vi "Global_Drive_Turn_sens.vi"() -> ()   [LabVIEW 2017]
panel:
  in  "Height Gear Max Turn Sens":dbl
  in  "Low Gear Max Turn Sens":dbl
  in  "Height Gear Min Turn Sens":dbl
  in  "Low Gear Min Turn Sens":dbl
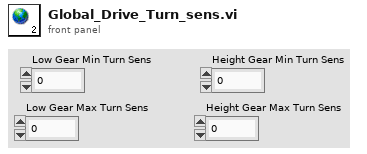
[diagram p1: front panel]
diagram:
